vi "GetType.vi"(8 "error in (no error)":errorcluster, 11 "Send Software Trigger Msg":refnum<class "Send Software Trigger Msg.lvclass">) -> (0 "error out":errorcluster, 2 "Data Sample":variant, 3 "Send Software Trigger Msg":refnum<class "Send Software Trigger Msg.lvclass">)   [LabVIEW 2015, in "CS++DMM.lvlib" / "Send Software Trigger Msg.lvclass"]
uses:
  Send Software Trigger Msg.lvclass
  Send Software Trigger Msg.lvclass/Send Software Trigger Msg.ctl
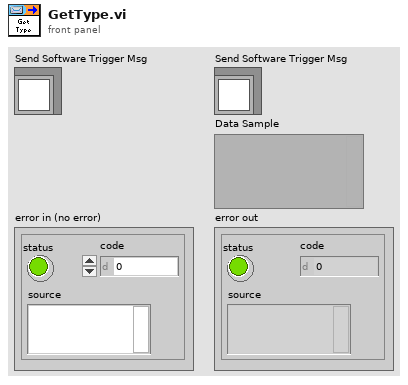
[diagram p1: front panel]
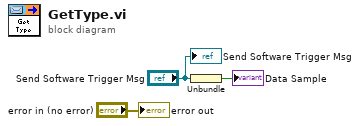
[diagram p0: block diagram]
diagram:
  n1 = Unbundle("Send Software Trigger Msg") -> (→"Data Sample":bool)
  "error out" <- "error in (no error)"
  "Send Software Trigger Msg" <- "Send Software Trigger Msg"
